vi "Listener VI.vi"(7 "Operation":T1, 8 "error in (no error)":errorcluster, 11 "Listener.lvclass":refnum<class "Listener.lvclass">) -> (0 "error out":errorcluster, 3 "Listener Out.lvclass":refnum<class "Listener.lvclass">)   [LabVIEW 2019]
doc: "Reads/Writes data using the specified protocol.\nInput: \nListener Object\nMessage: The \"packet\" which will be sent through the selected protocol\nOpeartion: Read/Write operation on the specified protocol\nAK?: Special parameter for AK TCP and RS-xxx protocol"
uses:
  Listener.lvclass
  ListenerClassControls/Operation Ctl.ctl
panel:
  in  "Message":string
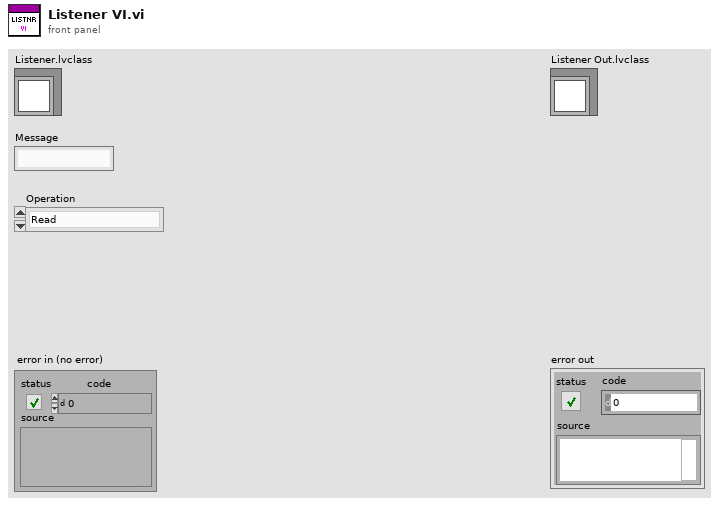
[diagram p1: front panel]
types:
  T1 = typedef "Operation Ctl.ctl" = enum16{"Read", "Write"}
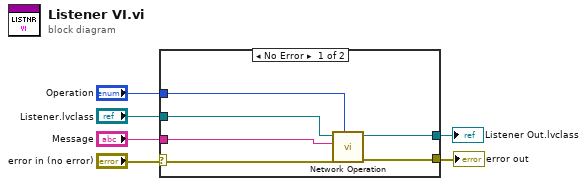
[diagram p0: block diagram]
diagram:
  n1 = case shown="No Error" "error in (no error)" {
    selector: "error in (no error)" -> [w9 w13]
    tunnel: "Listener.lvclass" -> [w12 w14]
    tunnel: [w11 w13] -> w6
    tunnel: [w10 w14] -> w5
    tunnel: "Operation" -> [w8 _]
    tunnel: "Message" -> [w7 _]
    frame No Error {
      n2 = call "Network Operation.vi"("Operation"=w8, "error in (no error)"=w9, "Message"=w7, "Listener In.lvclass"=w12) -> ("error out"=w11:errorcluster, "Listener Out.lvclass"=w10:refnum<class "Listener.lvclass">)  [unwired: 6 in]
    }
    frame Error {
    }
  }
  "error out" <- w6
  "Listener Out.lvclass" <- w5
